vi "Gain.vi"(11 "数组":dbl[](array[numeric])) -> (3 "K0":dbl)   [LabVIEW 2019]
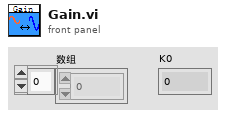
[diagram p1: front panel]
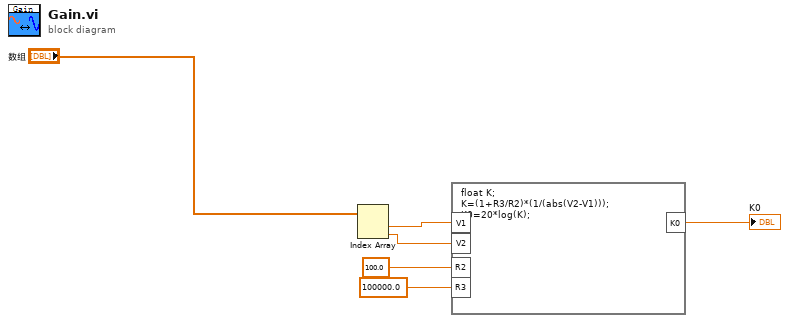
[diagram p0: block diagram]
diagram:
  n1 = Index Array(array="数组") -> (element #1=w6:dbl, element #2=w5:dbl)  [unwired: 2 in]
  n2 = formula code="float K;\nK=(1+R3/R2)*(1/(abs(V2-V1)));\nK0=20*log(K);"("V1"=w6, "V2"=w5, "R2"=100.0 ("输入变量"), "R3"=100000.0 ("输入变量")) -> ("K0"=→"K0":dbl)
